vi "Sous-VI_zone_securite2.vi"(2 "Coordonnées des drônes":T1, 3 "constante ii 2":errorcluster caption="constante d'erreur", 6 "Coordonnées du rectangle":T2) -> (16 "Booléen":bool, 17 "constante d'erreur":errorcluster)   [LabVIEW 2013]
panel:
  # "Ce sous-VI sert à indiquer la présence d'un drone dans la zone de sécurité (rectangle grisé).\nEn cas de présence, ce sous-VI renvoie un booléen \"1\" et en cas d'absence de drône dans la zone,\nle sous-VI renvoie \"0\"."
  # "Le cluster contenant les coordonnées du rectangle (respectivement les bords Gauche, Haut, Droite et Bas) est désassemblé,\nle cluster contenant les coordonnées des drônes également.\nPour qu'un drone soit dans la zone, il faut que son abscisse soit supérieure à la valeur du bord gauche du rectangle, inférieure au brod droit. Et son ordonnée doit être supérieure au bord haut du rectangle, inférieure au bord bas. Tous les comparateurs testent ces conditions. Ces 4 conditions doivent toutes être vérifiées, c'est pourquoi nous utilisons des portes \"ET\". Un seul des drones dans la zone suffit à renvoyer la valeur \"1\", c'est pourquoi nous utilisons des portes \"OU\"."
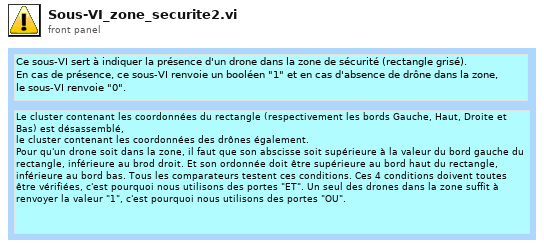
[diagram p1: front panel]
types:
  T1 = cluster{cluster{"X1 vert":i32, "Y1 vert":i32}, cluster{"X2 vert":i32, "Y2 vert":i32}, cluster{"X1 rouge":i32, "Y1 rouge":i32}, cluster{"X2 rouge":i32, "Y2 rouge":i32}}
  T2 = cluster{"Width":u16, "Width 2":u16, "Width 3":u16, "Width 4":u16}
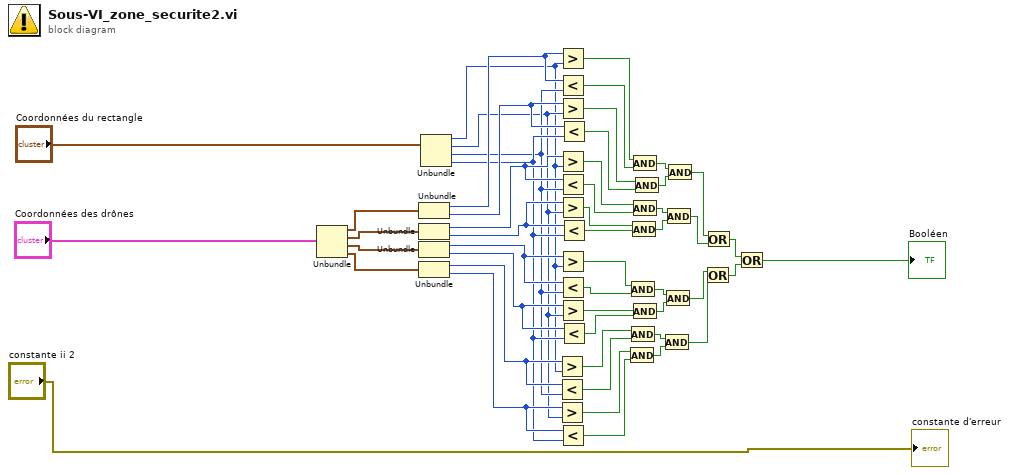
[diagram p0: block diagram]
diagram:
  n1 = Unbundle("Coordonnées des drônes") -> (w4:cluster{"X1 vert":i32, "Y1 vert":i32}, w3:cluster{"X2 vert":i32, "Y2 vert":i32}, w2:cluster{"X1 rouge":i32, "Y1 rouge":i32}, w1:cluster{"X2 rouge":i32, "Y2 rouge":i32})
  n2 = Unbundle(w4) -> ("X1 vert"=w43:i32, "Y1 vert"=w44:i32)
  n3 = Unbundle(w3) -> ("X2 vert"=w45:i32, "Y2 vert"=w46:i32)
  n4 = Unbundle(w2) -> ("X1 rouge"=w47:i32, "Y1 rouge"=w48:i32)
  n5 = Unbundle(w1) -> ("X2 rouge"=w49:i32, "Y2 rouge"=w50:i32)
  n6 = Unbundle("Coordonnées du rectangle") -> ("Width"=w23:u16, "Width 2"=w24:u16, "Width 3"=w25:u16, "Width 4"=w26:u16)
  n7 = Greater?(x=w49, y=w23) -> (0:w39:bool)
  n8 = Less?(x=w49, y=w25) -> (x < y?=w40:bool)
  n9 = Greater?(x=w50, y=w24) -> (0:w41:bool)
  n10 = Greater?(x=w43, y=w23) -> (0:w27:bool)
  n11 = Less?(x=w43, y=w25) -> (x < y?=w28:bool)
  n12 = Greater?(x=w44, y=w24) -> (0:w29:bool)
  n13 = Greater?(x=w45, y=w23) -> (0:w31:bool)
  n14 = Less?(x=w45, y=w25) -> (x < y?=w32:bool)
  n15 = Greater?(x=w46, y=w24) -> (0:w33:bool)
  n16 = Greater?(x=w47, y=w23) -> (0:w35:bool)
  n17 = Less?(x=w47, y=w25) -> (x < y?=w36:bool)
  n18 = Greater?(x=w48, y=w24) -> (0:w37:bool)
  n19 = Less?(x=w50, y=w26) -> (x < y?=w42:bool)
  n20 = Less?(x=w44, y=w26) -> (x < y?=w30:bool)
  n21 = Less?(x=w46, y=w26) -> (x < y?=w34:bool)
  n22 = Less?(x=w48, y=w26) -> (x < y?=w38:bool)
  n23 = And(x=w41, y=w42) -> (x .and. y?=w20:bool)
  n24 = And(x=w35, y=w36) -> (x .and. y?=w17:bool)
  n25 = And(x=w39, y=w40) -> (x .and. y?=w19:bool)
  n26 = And(x=w33, y=w34) -> (x .and. y?=w15:bool)
  n27 = And(x=w27, y=w28) -> (x .and. y?=w11:bool)
  n28 = And(x=w31, y=w32) -> (x .and. y?=w14:bool)
  n29 = And(x=w37, y=w38) -> (x .and. y?=w18:bool)
  n30 = And(x=w29, y=w30) -> (x .and. y?=w12:bool)
  n31 = And(x=w19, y=w20) -> (x .and. y?=w22:bool)
  n32 = And(x=w17, y=w18) -> (x .and. y?=w21:bool)
  n33 = And(x=w14, y=w15) -> (x .and. y?=w16:bool)
  n34 = And(x=w11, y=w12) -> (x .and. y?=w13:bool)
  n35 = Or(x=w21, y=w22) -> (x .or. y?=w8:bool)
  n36 = Or(x=w13, y=w16) -> (x .or. y?=w7:bool)
  n37 = Or(x=w7, y=w8) -> (x .or. y?=→"Booléen":bool)
  "constante d'erreur" <- "constante ii 2"
